vi "TH260_LibVersion_global.vi"() -> ()   [LabVIEW 2010]
panel:
  in  "Library Version":string="3.2"
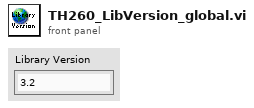
[diagram p1: front panel]
diagram:
